vi "zad1.vi"() -> ()   [LabVIEW 2017]
panel:
  in  "stop":bool
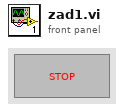
[diagram p1: front panel]
types:
  T1 = typedef "LVPositionTypeDef.ctl" = cluster{"Left":i32, "Top":i32}
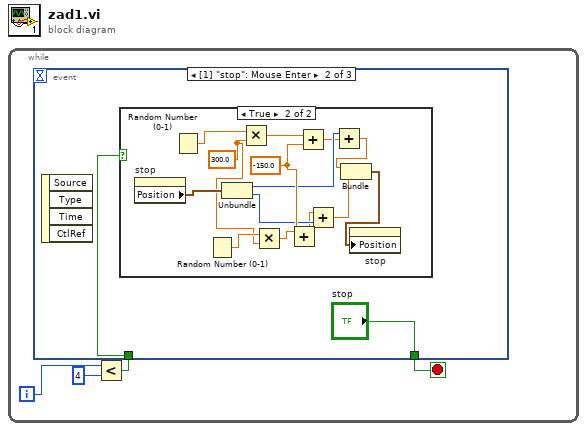
[diagram p0: block diagram]
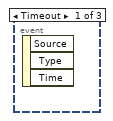
[diagram p2: hidden frame]
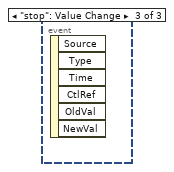
[diagram p4: hidden frame]
diagram:
  n1 = while {
    i -> [w3]
    stop <- w4 stop-if-true
    n2 = Less?(x=w3, y=4) -> (x < y?=w1:bool)
    n3 = event shown="[1] \"stop\": Mouse Enter" {
      selector: _ -> [_ _ _]
      dyn-events: _ -> [_ _ _]
      timeout: _ -> [_ _ _]
      tunnel: [_ "stop" _] -> w4
      tunnel: w1 -> [_ w5 _]
      event Timeout {
        n4 = event-data() -> ()  [unwired: 1 in, 3 out]
      }
      event "stop": Mouse Enter {
        n5 = event-data() -> ()  [unwired: 1 in, 4 out]
        n6 = case shown="True" w5 {
          frame False {
          }
          frame True {
            w14 = -150.0 ("y")
            w16 = 300.0 ("y")
            n7 = property on="stop" class="Bool"() -> ("Position"=w20:T1)  [unwired: 2 in, 2 out]
            n8 = Random Number (0-1)() -> (number: 0 to 1=w18:dbl)
            n9 = Random Number (0-1)() -> (number: 0 to 1=w17:dbl)
            n10 = Unbundle(w20) -> ("Left"=w12:i32, "Top"=w13:i32)
            n11 = Multiply(x=w18, y=w16) -> (x*y=w19:dbl)
            n12 = Multiply(x=w17, y=w16) -> (x*y=w15:dbl)
            n13 = Add(x=w15, y=w14) -> (x+y=w10:dbl)
            n14 = Add(x=w19, y=w14) -> (x+y=w11:dbl)
            n15 = Add(x=w10, y=w13) -> (x+y=w9:dbl)
            n16 = Add(x=w12, y=w11) -> (x+y=w8:dbl)
            n17 = Bundle(w8, w9) -> (w7:cluster{dbl, dbl})  [unwired: 1 in]
            n18 = property on="stop" class="Bool"("Position"=w7) -> ()  [unwired: 2 in, 2 out]
          }
        }
      }
      event "stop": Value Change {
        n19 = event-data() -> ()  [unwired: 1 in, 6 out]
      }
    }
  }
